vi "Read FPGA VI Reference Out.vi"(8 "error in (no error)":errorcluster, 11 "FPGASession in":refnum<class "FPGASession.lvclass">) -> (0 "error out":errorcluster, 2 "FPGA Interface":T1, 3 "FPGASession out":refnum<class "FPGASession.lvclass">)   [LabVIEW 2013, in "FPGASession.lvclass"]
uses:
  FPGASession.lvclass
  RT/FPGASession/FPGARef.ctl
  FPGASession.lvclass/FPGASession.ctl
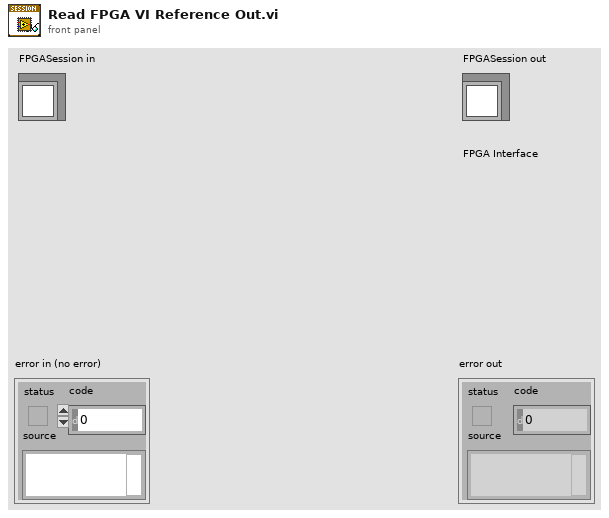
[diagram p1: front panel]
types:
  T1 = typedef "FPGASession.lvclass/FPGARef.ctl" = refnum<k20>
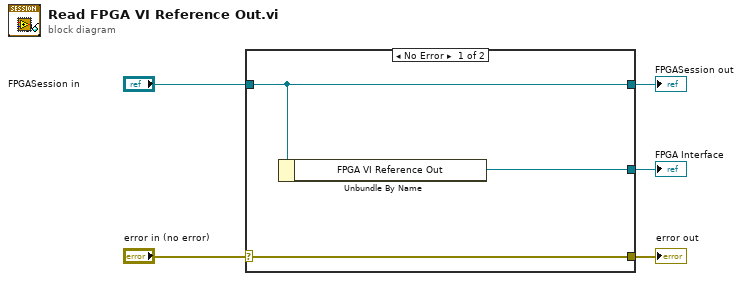
[diagram p0: block diagram]
diagram:
  n1 = case shown="No Error" "error in (no error)" {
    selector: "error in (no error)" -> [w8 w9]
    tunnel: [w8 w9] -> w4
    tunnel: [w7 w10] -> w2
    tunnel: "FPGASession in" -> [w7 w10]
    tunnel: [w6 _] -> w1
    frame No Error {
      n2 = Unbundle By Name(w7) -> ("FPGA VI Reference Out"=w6:T1)
    }
    frame Error {
    }
  }
  "error out" <- w4
  "FPGASession out" <- w2
  "FPGA Interface" <- w1
